vi "Interface_Asset_Update Tags.vi"(8 "error in (no error)":errorcluster, 10 "TagBus DVR":refnum<data-value>, 11 "Asset_Interface in":refnum<class "Load.lvclass">) -> (0 "error out":errorcluster, 2 "TagBus DVR out":refnum<data-value>, 3 "Asset_Interface out":refnum<class "Load.lvclass">)   [LabVIEW 2015, in "Load.lvclass"]
uses:
  Load.lvclass
  TagBus/TagBus.lvclass
  Load.lvclass/Load.ctl
panel:
  out "Status":cluster{"kW":dbl}
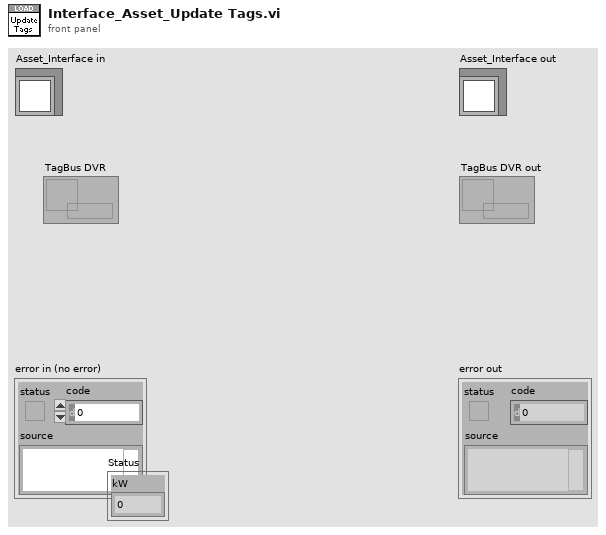
[diagram p1: front panel]
types:
  T1 = typedef "Load.lvclass/Load_Status.ctl" = cluster{"kW":dbl}
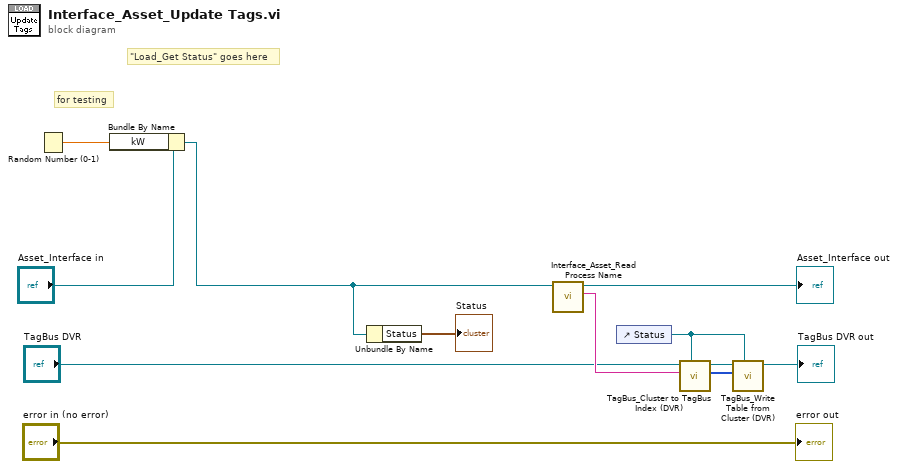
[diagram p0: block diagram]
diagram:
  # "\"Load_Get Status\" goes here"
  # "for testing"
  n1 = Random Number (0-1)() -> (number: 0 to 1=w10:dbl)
  n2 = Bundle By Name(cluster="Asset_Interface in", "kW"=w10) -> (w11:refnum<class "Load.lvclass">)
  n3 = Unbundle By Name(w11) -> ("Status"=→"Status":T1)
  n4 = call-dynamic "Interface_Asset_Read Process Name.vi"("Load in"=w11) -> ("Process Name"=w6:string, "Load out"=→"Asset_Interface out":refnum<class "Load.lvclass">)  [unwired: 9 in]
  n5 = control-ref of="Status"() -> (w7:refnum<vi>)
  n6 = call "TagBus_Cluster to TagBus Index (DVR).vi"("Clust Refnum"=w7, "Tag Name Prepend"=w6, "TagBus DVR"="TagBus DVR") -> ("Index Array"=w8:i32[], "TagBus DVR out"=w9:refnum<data-value>)  [unwired: 7 in]
  n7 = call "TagBus_Write Table from Cluster (DVR).vi"("Clust Refnum"=w7, "Index Array"=w8, "Data Value Reference in"=w9) -> ("Data Value Reference out"=→"TagBus DVR out":refnum<data-value>)  [unwired: 8 in]
  "error out" <- "error in (no error)"
